vi "QSM - Get Next State.vi"(6 "QSM":T1={"Invalid Option"=enum."Ignore", "QSM"=refnum}, 8 "error in (no error)":errorcluster) -> (0 "error out":errorcluster, 3 "State":string, 4 "Stop?":bool)   [LabVIEW 2014]
doc: "This VI Gets the next State.\nIf no state is enqueued, the QSM goes to the Idle State (Event Check)\nIf an error occurs, the QSM goes to the Error Handler State\nIf the VI Stop State is enqueued, the QSM is stopped\n\nDataEtc Copyright (c) 2013"
uses:
  TypeDef/QSM - STYP.ctl
  TypeDef/Invalid Option - STYP.ctl
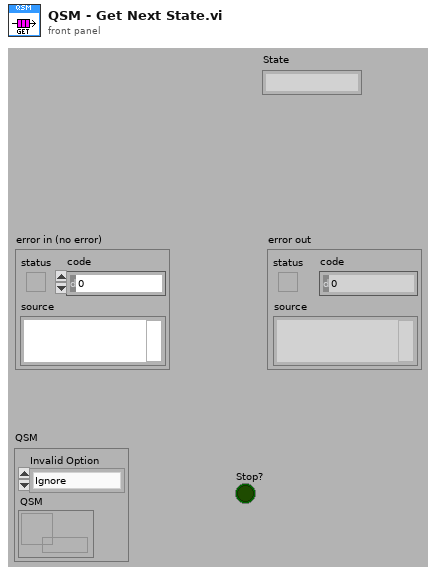
[diagram p1: front panel]
types:
  T1 = typedef "QSM - STYP.ctl" = cluster{"Invalid Option":T2, "QSM":refnum<queue>}
  T2 = typedef "Invalid Option - STYP.ctl" = enum16{"Dialog", "Error", "Ignore"}
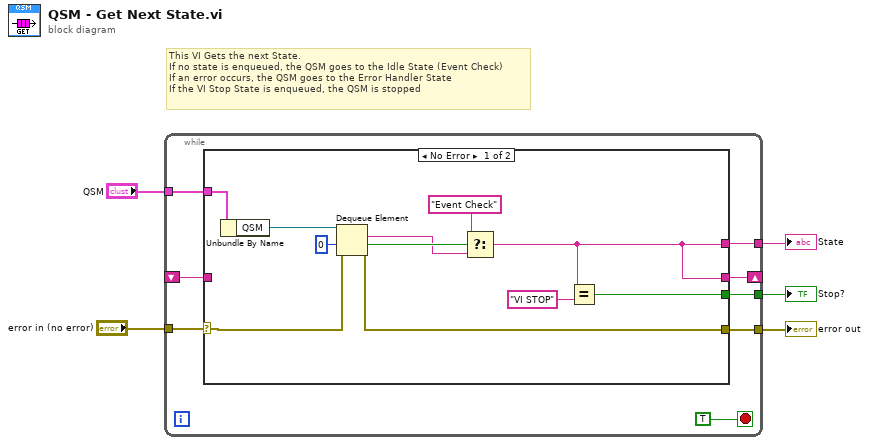
[diagram p0: block diagram]
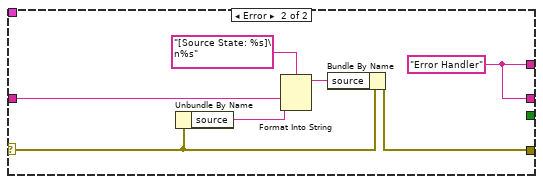
[diagram p2: hidden frame]
diagram:
  # "This VI Gets the next State.\nIf no state is enqueued, the QSM goes to the Idle State (Event Check)\nIf an error occurs, the QSM goes to the Error Handler State\nIf the VI Stop State is enqueued, the QSM is stopped"
  n1 = while {
    tunnel: "error in (no error)" -> [w12]
    tunnel: "QSM" -> [w11]
    tunnel: [w10] -> w3
    tunnel: [w9] -> w2
    shift-right: [w8] -> _
    shift-left: _ -> [w7]
    tunnel: [w6] -> w1
    stop <- TRUE stop-if-true
    n2 = case shown="No Error" w12 {
      selector: w12 -> [w22 w26]
      tunnel: w11 -> [w24 _]
      tunnel: [w21 w25] -> w10
      tunnel: [w16 w31] -> w9
      tunnel: [w16 w31] -> w8
      tunnel: w7 -> [_ w29]
      tunnel: [w14 _] -> w6
      frame No Error {
        n3 = Unbundle By Name(w24) -> ("QSM"=w23:refnum<queue>)
        n4 = Dequeue Element(queue=w23, timeout in ms (-1)=0, error in (no error)=w22) -> (element=w18:string, timed out?=w19:bool, error out=w21:errorcluster)  [unwired: 1 out]
        n5 = Select(t="Event Check", s=w19, f=w18) -> (s? t:f=w16:string)
        n6 = Equal?(x=w16, y="VI STOP") -> (x = y?=w14:bool)
      }
      frame Error {
        w31 = "Error Handler" ("t")
        n7 = Unbundle By Name(w26) -> ("source"=w28:string)
        n8 = Format Into String(format string="[Source State: %s]\n%s", w29, w28) -> (resulting string=w27:string)  [unwired: 2 in, 1 out]
        n9 = Bundle By Name(cluster=w26, "source"=w27) -> (w25:errorcluster)
      }
    }
  }
  "error out" <- w3
  "State" <- w2
  "Stop?" <- w1
